vi "s6.vi"() -> ()   [LabVIEW 2024]
panel:
  out "Waveform Graph":cluster{i32, i32, dbl[]}(graph)
  out "Iteration":dbl
  out "Current point":dbl
  in  "Points":u32
  in  "Range":u32
  in  "ActiveX Container":refnum<k7>(container)
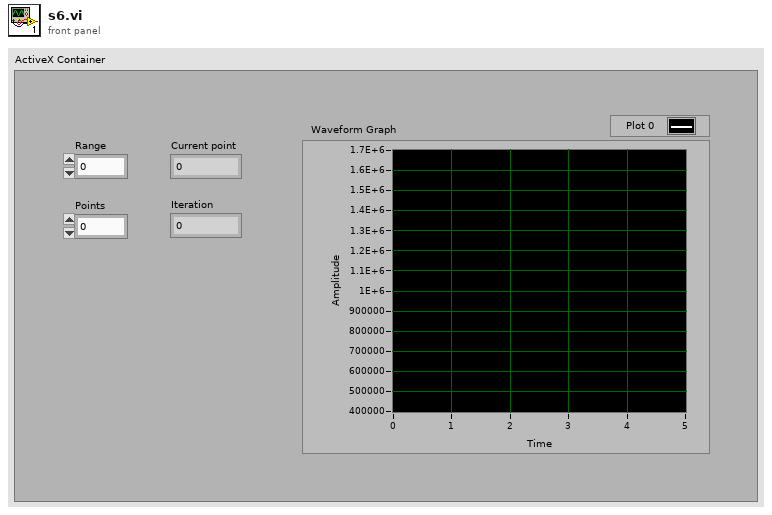
[diagram p1: front panel]
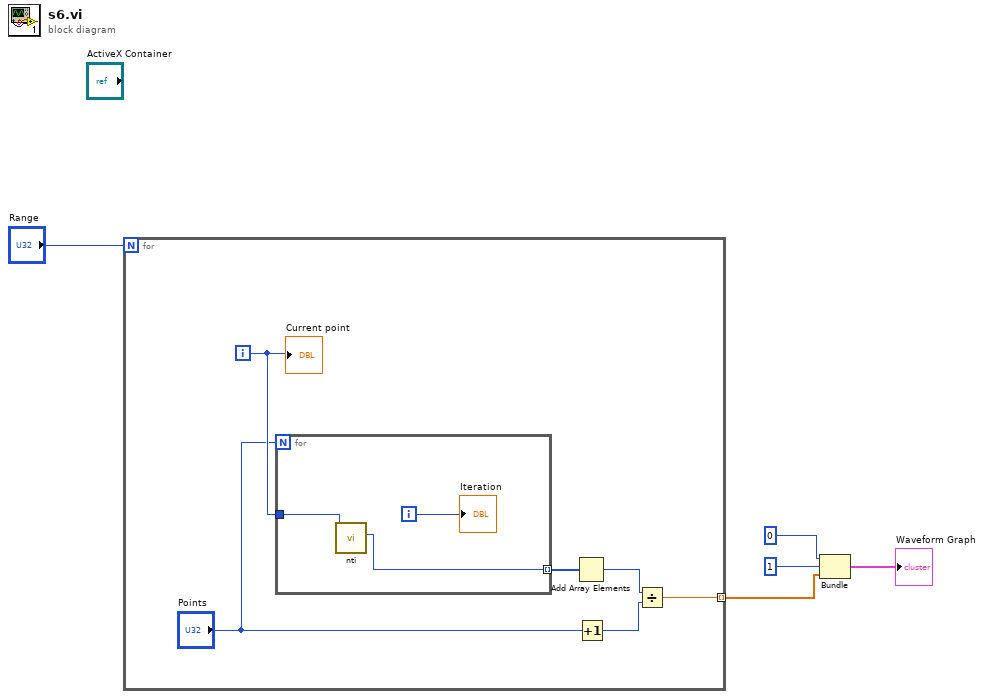
[diagram p0: block diagram]
diagram:
  n1 = for {
    N: "Range" -> [_]
    tunnel: [w8] -> w2 mode=indexing
    i -> [w11]
    n2 = for {
      N: "Points" -> [_]
      tunnel: w11 -> [w13]
      tunnel: [w12] -> w6 mode=indexing
      i -> [w14]
      n3 = call "nti.vi"("Number to match"=w13) -> ("Iterations"=w12:u32)  [unwired: 9 in, 1 out]
      "Iteration" <- w14
    }
    n4 = Add Array Elements(numeric array=w6) -> (sum=w10:u32)
    n5 = Increment(x="Points") -> (x+1=w9:u32)
    n6 = Divide(x=w10, y=w9) -> (x/y=w8:dbl)
    "Current point" <- w11
  }
  n7 = Bundle(0, 1, w2) -> (→"Waveform Graph":cluster{i32, i32, dbl[]})  [unwired: 1 in]
